vi "Calculate Tardiness (Prins FIFO Engine).vi"(8 "error in (no error)":errorcluster, 9 "Reorder?":bool, 10 "Schedule In":u16[](array[numeric]), 11 "OSSP_Problem in":refnum<class "OSSP_Problem.lvclass">) -> (0 "error out":errorcluster, 1 "Tardiness(Prins FIFO Engine)":u16, 2 "Schedule Out":u16[](array[numeric]), 3 "OSSP_Problem out":refnum<class "OSSP_Problem.lvclass">, 4 "Job Completion Times":i32[](array[numeric]))   [LabVIEW 2013, in "Scheduler.lvclass"]
uses:
  Scheduler.lvclass
  OSSP_Problem.lvclass
  OSSP_Problem.lvclass/OSSP_Problem.ctl
  UpdateMachineGaps.vi
  UpdateJobGaps.vi
  Find Intersecting Gaps.vi
  Transform to Plain Job and Machine Gaps Array.vi
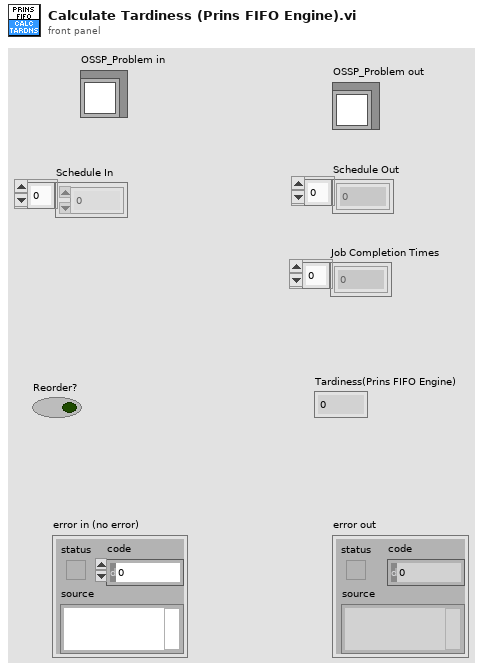
[diagram p1: front panel]
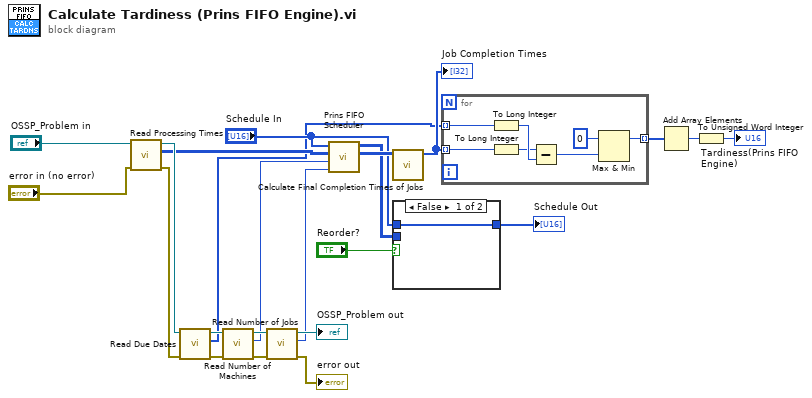
[diagram p0: block diagram]
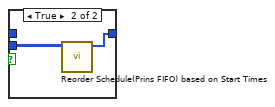
[diagram p2: hidden frame]
diagram:
  n1 = call "Read Processing Times.vi"("error in (no error)"="error in (no error)", "OSSP_Problem in"="OSSP_Problem in") -> ("error out"=w10:errorcluster, "Processing Times"=w4:u16[][], "OSSP_Problem out"=w13:refnum<class "OSSP_Problem.lvclass">)  [unwired: 7 in]
  n2 = call "Read Due Dates.vi"("error in (no error)"=w10, "OSSP_Problem in"=w13) -> ("error out"=w9:errorcluster, "Due Dates"=w3:u16[], "OSSP_Problem out"=w12:refnum<class "OSSP_Problem.lvclass">)  [unwired: 7 in]
  n3 = call "Read Number of Machines.vi"("error in (no error)"=w9, "OSSP_Problem in"=w12) -> ("error out"=w8:errorcluster, "Number of Machines"=w2:i32, "OSSP_Problem out"=w11:refnum<class "OSSP_Problem.lvclass">)  [unwired: 7 in]
  n4 = call "Read Number of Jobs.vi"("error in (no error)"=w8, "OSSP_Problem in"=w11) -> ("error out"=→"error out":errorcluster, "Number of Jobs"=w1:i32, "OSSP_Problem out"=→"OSSP_Problem out":refnum<class "OSSP_Problem.lvclass">)  [unwired: 7 in]
  n5 = call "Prins FIFO Scheduler.vi"("Number of Jobs"=w1, "Number of Machines"=w2, "Processing Times(MxJ)"=w4, "Schedule In"="Schedule In") -> ("Completion Times (MxJ)"=w20:i32[][], "Start Times (MxJ)"=w18:i32[][])  [unwired: 6 in]
  n6 = call "Calculate Final Completion Times of Jobs.vi"("Completion Times (MxJ)"=w20) -> ("Job Completion Times"=w19:i32[])  [unwired: 10 in]
  "Job Completion Times" <- w19
  n7 = case shown="False" "Reorder?" {
    tunnel: w18 -> [_ w26]
    tunnel: [w24 w25] -> w17
    tunnel: "Schedule In" -> [w24 _]
    frame False {
    }
    frame True {
      n8 = call "Reorder Schedule(Prins FIFO) based on Start Times.vi"("Start Times (MxJ)"=w26) -> ("Reordered Schedule(Prins FIFO)"=w25:u16[])  [unwired: 10 in]
    }
  }
  "Schedule Out" <- w17
  n9 = for {
    tunnel: w3 -> [w33] mode=indexing
    tunnel: [w28] -> w23 mode=indexing
    tunnel: w19 -> [w27] mode=indexing
    n10 = To Long Integer(number=w33) -> (32bit integer=w32:i32)
    n11 = To Long Integer(number=w27) -> (32bit integer=w31:i32)
    n12 = Subtract(x=w31, y=w32) -> (x-y=w30:i32)
    n13 = Max & Min(x=0, y=w30) -> (max(x,y)=w28:i32)  [unwired: 1 out]
  }
  n14 = Add Array Elements(numeric array=w23) -> (sum=w22:i32)
  n15 = To Unsigned Word Integer(number=w22) -> (unsigned 16bit integer=→"Tardiness(Prins FIFO Engine)":u16)
